vi "RT Overlay Helper.vi"(11 "Refnum in":T1) -> (3 "Refnum out":T1)   [LabVIEW 2012]
uses:
  <vilib>/vision/Image Controls.llb/IMAQ Image.ctl
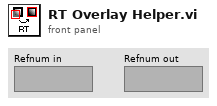
[diagram p1: front panel]
types:
  T1 = typedef "IMAQ Image.ctl" = refnum<image>
  T2 = typedef "Image Type" = u32
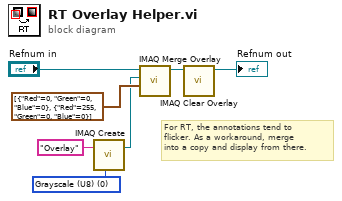
[diagram p0: block diagram]
diagram:
  w2 = T2 0 items=["Grayscale (U8)", "Grayscale (I16)", "Grayscale (SGL)", "Complex (CSG)", "RGB (U32)", "HSL (U32)", "RGB (U64)", "Grayscale (U16)"] ("Image Type")
  # "For RT, the annotations tend to\nflicker. As a workaround, merge\ninto a copy and display from there."
  n1 = call "IMAQ Create"("Image Name"="Overlay", "Image Type"=w2) -> ("New Image"=w6:T1)  [unwired: 2 in, 2 out]
  n2 = call "IMAQ Merge Overlay"("Color Palette"=cluster{"Red":u8, "Green":u8, "Blue":u8}[] [{"Red"=0, "Green"=0, "Blue"=0}, {"Red"=255, "Green"=0, "Blue"=0}], "Image Dst"=w6, "Image Src"="Refnum in") -> ("Image Dst Out"=w4:T1)  [unwired: 7 in, 1 out]
  n3 = call "IMAQ Clear Overlay"("Image"=w4) -> ("Image Out"=→"Refnum out":T1)  [unwired: 2 in, 8 out]
